vi "DIAG_TCP Check Connection.vi"(7 "Name":string, 8 "error in (no error)":errorcluster, 10 "ref in":T1, 11 "Connection In":T2) -> (0 "error out":errorcluster, 2 "Disconnected":bool, 3 "Connection out":T2)   [LabVIEW 2015, in "Diagnostics Addon Engine.lvlib"]
doc: "This VI removes the host connection from the connection manager list if it becomes disconnected for any reason."
uses:
  Diagnostics Addon Engine.lvlib
  TCP/stm_TCP Connection Info.ctl
  _SubVIs/stm_MetaDataElement.ctl
  STM Lookup Table Ref.ctl
  stm_TCPConnectionMethod.ctl
  <vilib>/NI Veristand/Custom Device Tools/Custom Device Utility Library/Custom Device Utility Library.lvlib
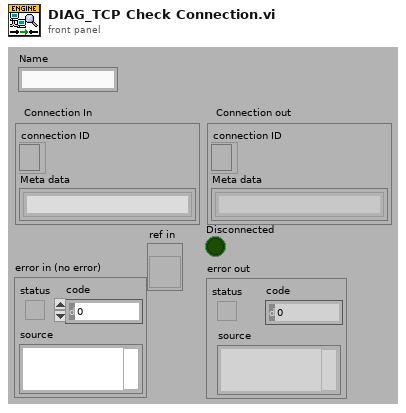
[diagram p1: front panel]
types:
  T1 = typedef "Diagnostics Addon Engine.lvlib/STM Lookup Table Ref.ctl" = refnum<vi>
  T2 = typedef "Diagnostics Addon Engine.lvlib/stm_TCP Connection Info.ctl" = cluster{"connection ID":refnum<k5>, "Meta data":T3[]}
  T3 = typedef "Diagnostics Addon Engine.lvlib/stm_MetaDataElement.ctl" = string
  T4 = typedef "Diagnostics Addon Engine.lvlib/stm_TCPConnectionMethod.ctl" = enum16{"Initialize", "Add Connection", "Set Properties", "Get Connection(s)", "Remove Connection", "Remove All Connections", "Get Connection Count"}
  T5 = typedef "Diagnostics Addon Engine.lvlib/stm_TCPConnectionProperties.ctl" = cluster{"Name":string, "Address":string, "Custom":string}
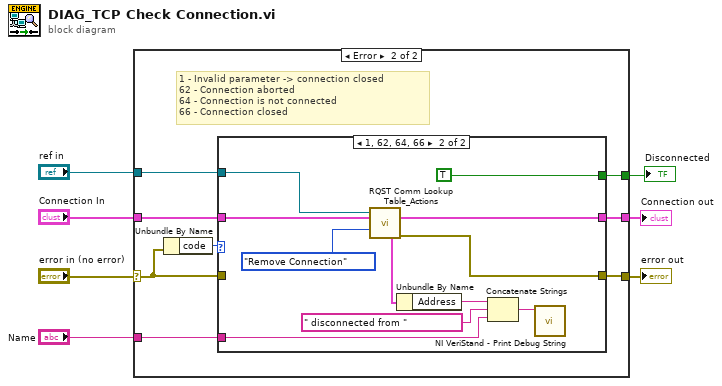
[diagram p0: block diagram]
diagram:
  n1 = case shown="Error" "error in (no error)" {
    selector: "error in (no error)" -> [w9 w16]
    tunnel: [w9 w15] -> w6
    tunnel: "Connection In" -> [w8 w14]
    tunnel: [w8 w13] -> w4
    tunnel: [_ w12] -> w3
    tunnel: "ref in" -> [_ w11]
    tunnel: "Name" -> [_ w10]
    frame No Error {
    }
    frame Error {
      # "1 - Invalid parameter -> connection closed\n62 - Connection aborted\n64 - Connection is not connected\n66 - Connection closed"
      n2 = Unbundle By Name(w16) -> ("code"=w17:i32)
      n3 = case shown="1, 62, 64, 66" w17 {
        tunnel: w16 -> [w19 _]
        tunnel: [w19 w27] -> w15
        tunnel: w14 -> [w18 w28]
        tunnel: [w18 w26] -> w13
        tunnel: [_ TRUE] -> w12
        tunnel: w11 -> [_ w25]
        tunnel: w10 -> [_ w20]
        frame 0, Default {
        }
        frame 1, 62, 64, 66 {
          n4 = call "RQST Comm Lookup Table_Actions.vi"("ref in"=w25, "Connection In"=w28, "Method"=stm_TCPConnectionMethod."Remove Connection") -> ("Connection Out"=w26:T2, "Properties Out"=w24:T5, "error out"=w27:errorcluster)  [unwired: 6 in, 4 out]
          n5 = Unbundle By Name(w24) -> ("Address"=w21:string)
          n6 = Concatenate Strings(w21, " disconnected from " ("string"), w20) -> (w23:string)
          n7 = call <vilib>:"NI VeriStand - Print Debug String.vi"("Message"=w23) -> ()  [unwired: 10 in, 1 out]
        }
      }
    }
  }
  "error out" <- w6
  "Connection out" <- w4
  "Disconnected" <- w3
